vi "Facade.vi"(0 "Data In":T5, 2 "Display State In":T3, 3 "Container State":T4) -> (6 "Data Out":T5, 7 "Display State Out":T3, 8 "Action":T2)   [LabVIEW 2020, in "Level XCtl.xctl"]
uses:
  Level XCtl.xctl
  Level Data.ctl
  Level Units.ctl
  <vilib>/_xctls/Container State.ctl
  State.ctl
  <vilib>/_xctls/Action.ctl
  <vilib>/_xctls/XControlSupport.lvlib
panel:
  out "Max":dbl
  in  "Mode":T1
  in  "Level":dbl
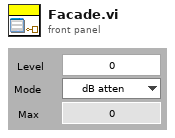
[diagram p1: front panel]
types:
  T1 = typedef "Level Units.ctl" = enum16{"dB atten", "dB SPL", "dB re 1 Vrms", "dB V/Hz½", "mW", "dB HL", "Volts", "dB mW"}
  T2 = typedef "XControlSupport.lvlib/Action.ctl" = cluster{"Data Changed?":bool, "State Changed?":bool, "Action Name":string}
  T3 = typedef "Level XCtl.xctl/State.ctl" = cluster{"Numeric":dbl}
  T4 = typedef "XControlSupport.lvlib/Container State.ctl" = cluster{"Indicator?":bool, "Run Mode?":bool, " Refnum":refnum<vi>}
  T5 = typedef "Level XCtl.xctl/Level Data.ctl" = cluster{"Level":dbl, "Units":T1, "Max":dbl, "Multiplier":dbl, "Cal File":path, "Cal":cluster{"Freq (Hz)":dbl[], "Mag (dB SPL)":dbl[], "Phase (deg)":dbl[]}}
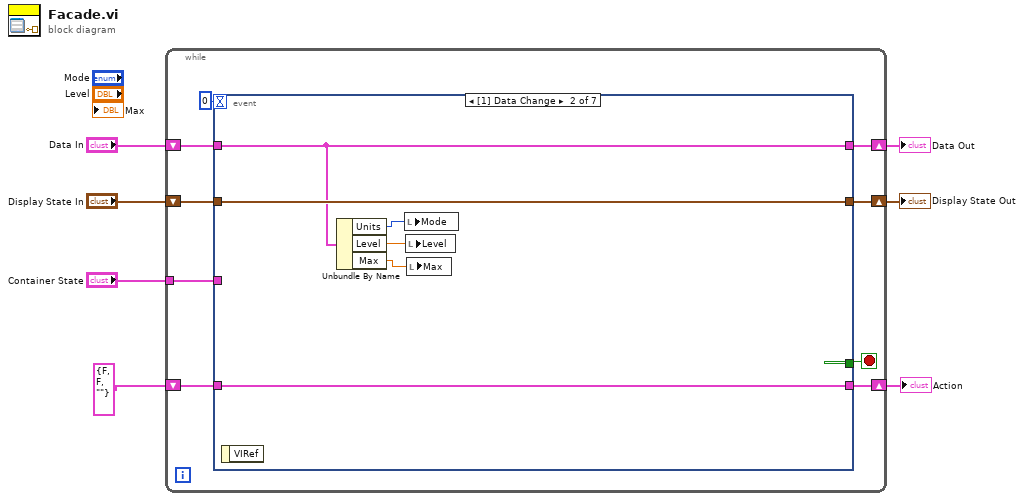
[diagram p0: block diagram]
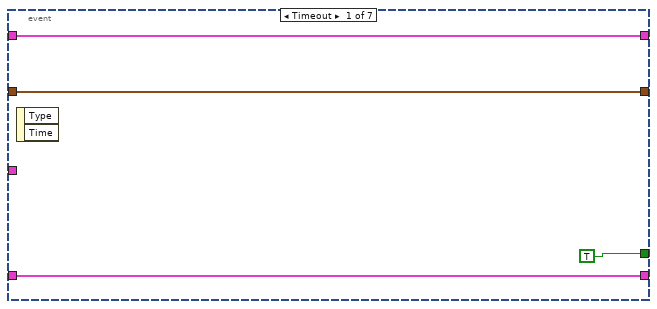
[diagram p2: hidden frame]
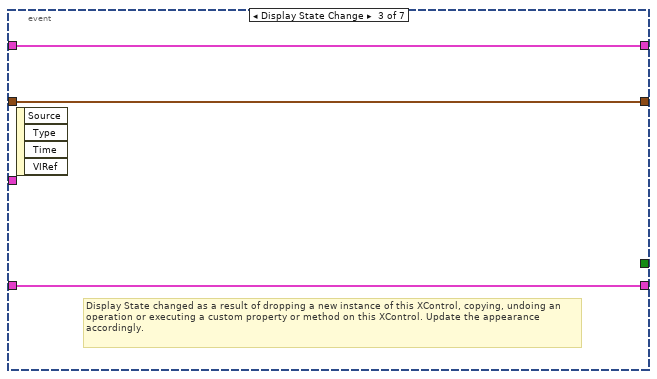
[diagram p3: hidden frame]
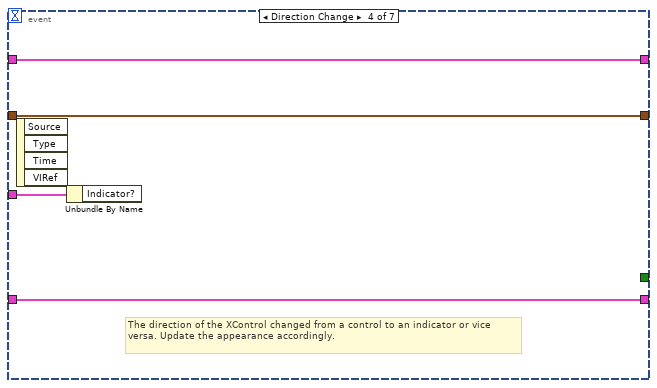
[diagram p4: hidden frame]
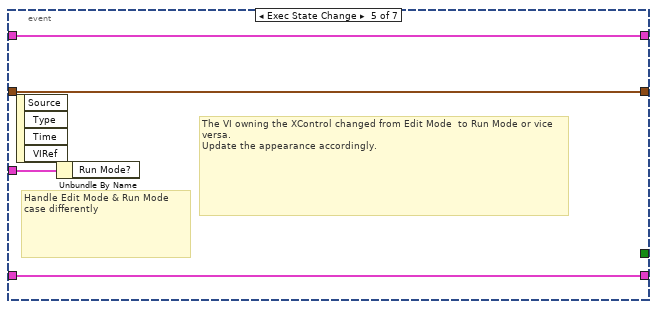
[diagram p5: hidden frame]
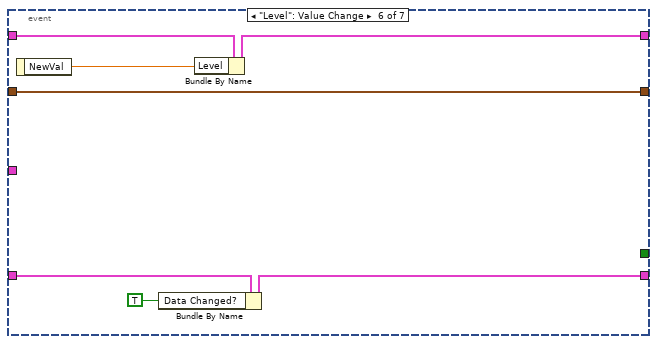
[diagram p6: hidden frame]
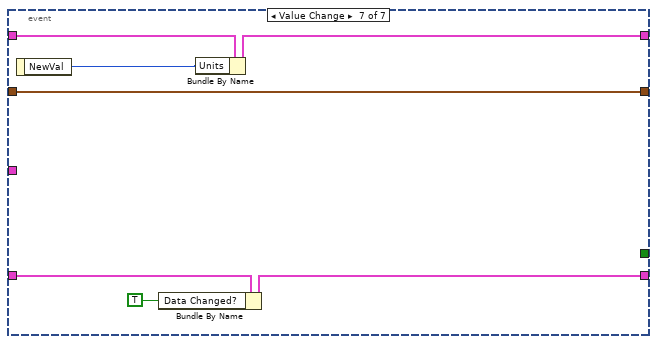
[diagram p7: hidden frame]
diagram:
  n1 = while {
    shift-right: [w15] -> w4
    shift-left: "Display State In" -> [w16]
    tunnel: "Container State" -> [w12]
    shift-right: [w10] -> w7
    shift-left: "Data In" -> [w11]
    shift-right: [w8] -> w2
    shift-left: T2 {"Data Changed?"=FALSE, "State Changed?"=FALSE, "Action Name"=""} ("Action") -> [w9]
    stop <- w14 stop-if-true
    n2 = event shown="[1] Data Change" {
      selector: _ -> [_ _ _ _ _ _ _]
      dyn-events: _ -> [_ _ _ _ _ _ _]
      timeout: 0 -> [_ _ _ _ _ _ _]
      tunnel: w16 -> [w18 w26 w29 w32 w36 w38 w45]
      tunnel: [w18 w26 w29 w32 w36 w38 w45] -> w15
      tunnel: [TRUE _ _ _ _ _ _] -> w14
      tunnel: w12 -> [_ _ _ w33 w37 _ _]
      tunnel: w11 -> [w17 w24 w28 w31 w35 w44 w51]
      tunnel: [w17 w24 w28 w31 w35 w42 w49] -> w10
      tunnel: [w19 w25 w27 w30 w34 w39 w46] -> w8
      tunnel: w9 -> [w19 w25 w27 w30 w34 w41 w48]
      event Timeout {
        n3 = event-data() -> ()  [unwired: 1 in, 2 out]
      }
      event Data Change {
        n4 = event-data() -> ()  [unwired: 1 in, 1 out]
        n5 = Unbundle By Name(w24) -> ("Units"=w22:T1, "Level"=w23:dbl, "Max"=w21:dbl)
        n6 = local write "Mode"(w22) -> ()
        n7 = local write "Level"(w23) -> ()
        n8 = local write "Max"(w21) -> ()
      }
      event Display State Change {
        # "Display State changed as a result of dropping a new instance of this XControl, copying, undoing an operation or executing a custom property or method on this XControl. Update the appearance accordingly."
        n9 = event-data() -> ()  [unwired: 1 in, 4 out]
      }
      event Direction Change {
        # "The direction of the XControl changed from a control to an indicator or vice versa. Update the appearance accordingly."
        n10 = event-data() -> ()  [unwired: 1 in, 4 out]
        n11 = Unbundle By Name(w33) -> ()  [unwired: 1 out]
      }
      event Exec State Change {
        # "The VI owning the XControl changed from Edit Mode  to Run Mode or vice versa.\nUpdate the appearance accordingly."
        # "Handle Edit Mode & Run Mode\ncase differently"
        n12 = event-data() -> ()  [unwired: 1 in, 4 out]
        n13 = Unbundle By Name(w37) -> ()  [unwired: 1 out]
      }
      event "Level": Value Change {
        n14 = event-data() -> ("NewVal"=w43:dbl)  [unwired: 1 in]
        n15 = Bundle By Name(cluster=w41, "Data Changed?"=TRUE) -> (w39:T2)
        n16 = Bundle By Name(cluster=w44, "Level"=w43) -> (w42:T5)
      }
      event Value Change {
        n17 = event-data() -> ("NewVal"=w50:T1)  [unwired: 1 in]
        n18 = Bundle By Name(cluster=w48, "Data Changed?"=TRUE) -> (w46:T2)
        n19 = Bundle By Name(cluster=w51, "Units"=w50) -> (w49:T5)
      }
    }
  }
  "Display State Out" <- w4
  "Data Out" <- w7
  "Action" <- w2
